vi "Initialize Max Allowed PDP Current Array.vi"(2 "error in":errorcluster, 3 "Robot ID":string="981") -> (0 "error out":errorcluster, 1 "output array":dbl[](array[numeric]))   [LabVIEW 2019]
panel:
  out "Post WLRA":dbl[](array[numeric])
  out "Post Drive Motors":dbl[](array[numeric])
  out "initialized array":dbl[](array[numeric])
  out "Max Allowed Current":i32
  out "PDP Channel ID":i32
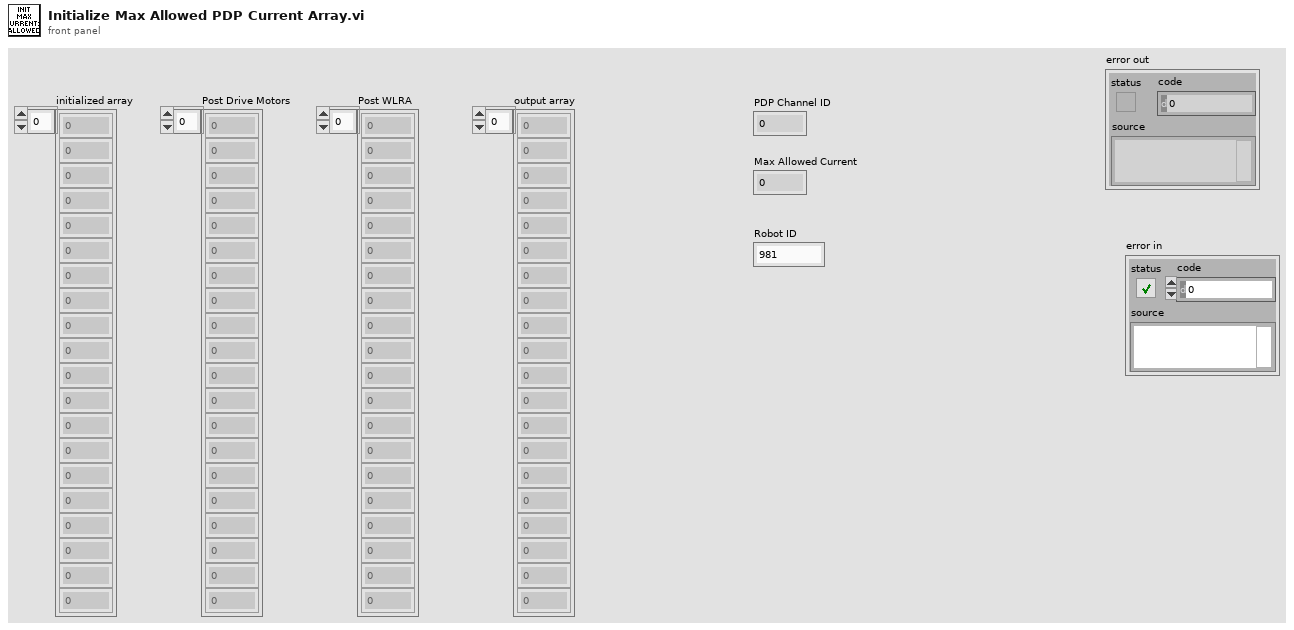
[diagram p1: front panel]
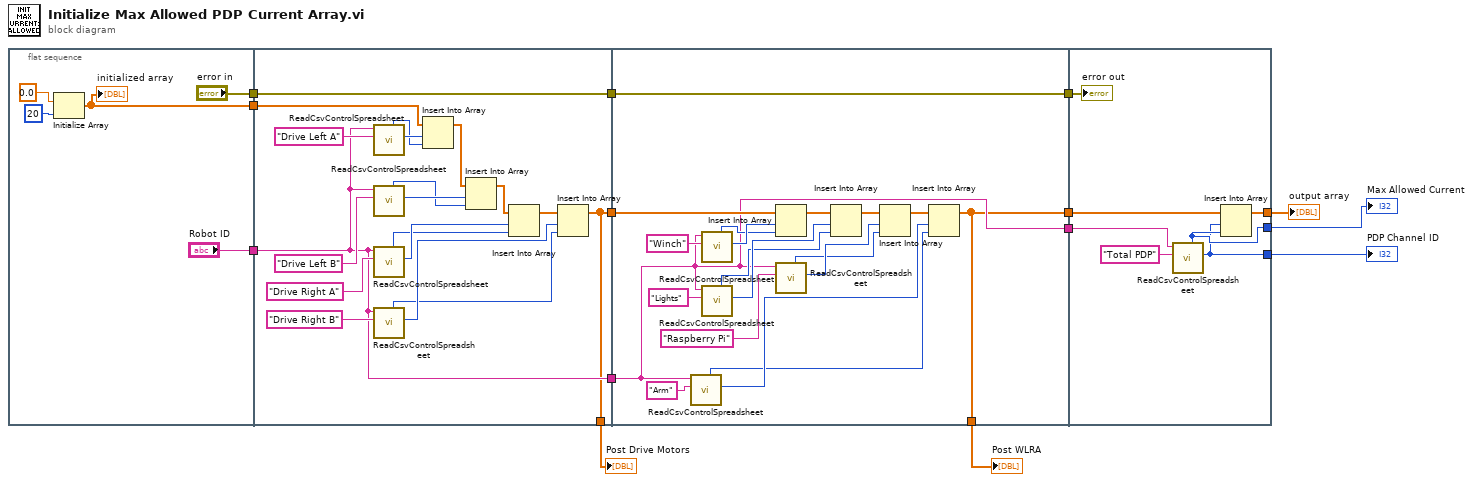
[diagram p0: block diagram]
diagram:
  n1 = flat-sequence {
    tunnel: [w17] -> w9
    tunnel: ["Robot ID"] -> w6
    tunnel: ["error in"] -> w3
    tunnel: w9 -> [w23]
    tunnel: [w20] -> w8
    tunnel: [w22] -> w7
    tunnel: w6 -> [w22]
    tunnel: [w21] -> w4
    tunnel: w3 -> [w21]
    tunnel: [w20] -> w2
    tunnel: [w39] -> w11
    tunnel: [w41] -> w10
    tunnel: w8 -> [w42]
    tunnel: w7 -> [w41]
    tunnel: [w40] -> w5
    tunnel: w4 -> [w40]
    tunnel: [w39] -> w1
    tunnel: [w63] -> w12
    tunnel: [w60] -> w13
    tunnel: [w59] -> w14
    tunnel: w11 -> [w64]
    tunnel: w10 -> [w61]
    tunnel: w5 -> [w58]
    frame #0 {
      n2 = Initialize Array(0.0 ("element"), 20 ("dimension size")) -> (w17:dbl[])
      "initialized array" <- w17
    }
    frame #1 {
      n3 = call "ReadCsvControlSpreadsheet.vi"("Motor ID"="Drive Left A", "Robot ID"=w22) -> ("PDP Channel ID"=w29:i32, "Max Allowed Current"=w27:i32)  [unwired: 1 in, 5 out]
      n4 = call "ReadCsvControlSpreadsheet.vi"("Motor ID"="Drive Left B", "Robot ID"=w22) -> ("PDP Channel ID"=w30:i32, "Max Allowed Current"=w26:i32)  [unwired: 1 in, 5 out]
      n5 = call "ReadCsvControlSpreadsheet.vi"("Motor ID"="Drive Right A", "Robot ID"=w22) -> ("PDP Channel ID"=w33:i32, "Max Allowed Current"=w25:i32)  [unwired: 1 in, 5 out]
      n6 = call "ReadCsvControlSpreadsheet.vi"("Motor ID"="Drive Right B", "Robot ID"=w22) -> ("PDP Channel ID"=w38:i32, "Max Allowed Current"=w24:i32)  [unwired: 1 in, 5 out]
      n7 = Insert Into Array(array=w23, index=w29, new element=w27) -> (w32:dbl[])
      n8 = Insert Into Array(array=w32, index=w30, new element=w26) -> (w35:dbl[])
      n9 = Insert Into Array(array=w35, index=w33, new element=w25) -> (w37:dbl[])
      n10 = Insert Into Array(array=w37, index=w38, new element=w24) -> (w20:dbl[])
    }
    frame #2 {
      n11 = call "ReadCsvControlSpreadsheet.vi"("Motor ID"="Arm", "Robot ID"=w41) -> ("PDP Channel ID"=w57:i32, "Max Allowed Current"=w43:i32)  [unwired: 1 in, 5 out]
      n12 = call "ReadCsvControlSpreadsheet.vi"("Motor ID"="Winch", "Robot ID"=w41) -> ("PDP Channel ID"=w48:i32, "Max Allowed Current"=w46:i32)  [unwired: 1 in, 5 out]
      n13 = call "ReadCsvControlSpreadsheet.vi"("Motor ID"="Lights", "Robot ID"=w41) -> ("PDP Channel ID"=w51:i32, "Max Allowed Current"=w45:i32)  [unwired: 1 in, 5 out]
      n14 = Insert Into Array(array=w42, index=w48, new element=w46) -> (w50:dbl[])
      n15 = call "ReadCsvControlSpreadsheet.vi"("Motor ID"="Raspberry Pi", "Robot ID"=w41) -> ("PDP Channel ID"=w54:i32, "Max Allowed Current"=w44:i32)  [unwired: 1 in, 5 out]
      n16 = Insert Into Array(array=w50, index=w51, new element=w45) -> (w52:dbl[])
      n17 = Insert Into Array(array=w52, index=w54, new element=w44) -> (w55:dbl[])
      n18 = Insert Into Array(array=w55, index=w57, new element=w43) -> (w39:dbl[])
    }
    frame #3 {
      n19 = call "ReadCsvControlSpreadsheet.vi"("Motor ID"="Total PDP", "Robot ID"=w61) -> ("PDP Channel ID"=w59:i32, "Max Allowed Current"=w60:i32)  [unwired: 1 in, 5 out]
      n20 = Insert Into Array(array=w64, index=w59, new element=w60) -> (w63:dbl[])
      "error out" <- w58
    }
  }
  "output array" <- w12
  "PDP Channel ID" <- w14
  "Max Allowed Current" <- w13
  "Post Drive Motors" <- w2
  "Post WLRA" <- w1
